vi "Get Configuration File Path.vi"() -> (3 "Configuration File Path":path)   [LabVIEW 2016, in "Assert API Components.lvlib"]
uses:
  Assert API Components/Assert API Components.lvlib
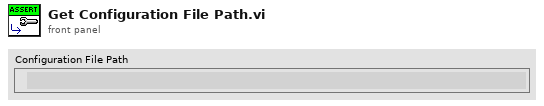
[diagram p1: front panel]
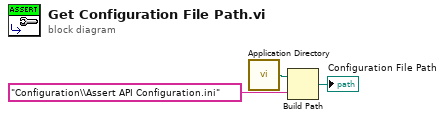
[diagram p0: block diagram]
diagram:
  n1 = call <vilib>:"Application Directory.vi"() -> ("Application Directory"=w2:path)
  n2 = Build Path(base path=w2, name or relative path="Configuration\\Assert API Configuration.ini") -> (appended path=→"Configuration File Path":path)
